vi "DIAdem Parameter CSC.vi"(4 "error in (no error)":errorcluster, 5 "Additional Parameter":string, 6 "Parameter":string, 7 "File Directory":path) -> (0 "error out":errorcluster, 3 "DIAdem Command Parameter":string)   [LabVIEW 2017]
doc: "This VI bundles special additional DIAdem start parameters."
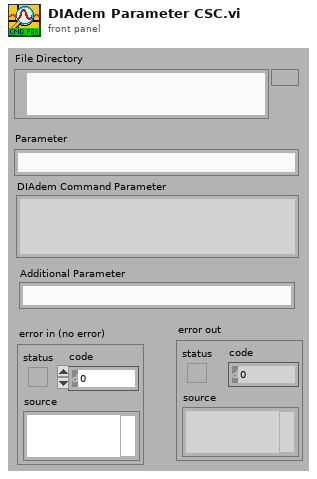
[diagram p1: front panel]
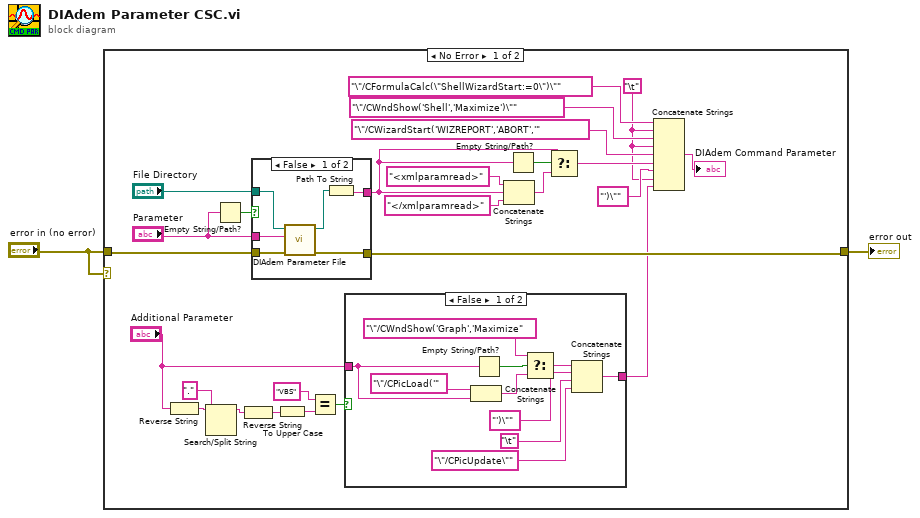
[diagram p0: block diagram]
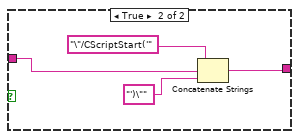
[diagram p2: hidden frame]
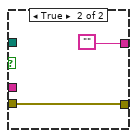
[diagram p3: hidden frame]
diagram:
  n1 = case shown="No Error" "error in (no error)" {
    tunnel: "error in (no error)" -> [w23 w51]
    tunnel: [w22 w51] -> w1
    frame No Error {
      w12 = "\t"
      n2 = Reverse String(1:"Additional Parameter") -> (0:w10:string)
      n3 = Search/Split String(string=w10, search string/char (-)="." ("search char (-)")) -> (substring before match=w9:string)  [unwired: 1 in, 2 out]
      n4 = Empty String/Path?(string/path="Parameter") -> (empty?=w20:bool)
      n5 = Reverse String(1:w9) -> (0:w8:string)
      n6 = case shown="False" w20 {
        tunnel: w23 -> [w48 w50]
        tunnel: [w47 w50] -> w22
        tunnel: "File Directory" -> [w46 _]
        tunnel: "Parameter" -> [w45 _]
        tunnel: [w43 ""] -> w18
        frame False {
          n7 = call <vilib>:"DIAdem Parameter File.vi"("error in (no error)"=w48, "Parameter"=w45, "File Directory"=w46) -> ("error out"=w47:errorcluster, "Parameter File"=w44:path)  [unwired: 3 in]
          n8 = Path To String(path=w44) -> (string=w43:string)
        }
        frame True {
        }
      }
      n9 = To Upper Case(1:w8) -> (0:w7:string)
      n10 = Equal?(x="VBS" ("Substring"), y=w7) -> (x = y?=w4:bool)
      n11 = case shown="False" w4 {
        tunnel: "Additional Parameter" -> [w34 w41]
        tunnel: [w29 w40] -> w3
        frame False {
          n12 = Concatenate Strings("\"/CPicLoad('" ("command"), w34) -> (w36:string)
          n13 = Empty String/Path?(string/path=w34) -> (empty?=w37:bool)
          n14 = Select(t="\"/CWndShow('Graph','Maximize", s=w37, f=w36) -> (s? t:f=w33:string)
          n15 = Concatenate Strings(w33, "')\"" ("Substring"), "\t", "\"/CPicUpdate\"" ("command")) -> (w29:string)
        }
        frame True {
          n16 = Concatenate Strings("\"/CScriptStart('" ("command"), w41, "')\"" ("Substring")) -> (w40:string)
        }
      }
      n17 = Concatenate Strings("<xmlparamread>", w18, "</xmlparamread>") -> (w27:string)
      n18 = Empty String/Path?(string/path=w18) -> (empty?=w26:bool)
      n19 = Select(t=w18, s=w26, f=w27) -> (s? t:f=w17:string)
      n20 = Concatenate Strings("\"/CFormulaCalc(\"ShellWizardStart:=0\")\"" ("DIAdem Command"), w12, "\"/CWndShow('Shell','Maximize')\"", w12, "\"/CWizardStart('WIZREPORT','ABORT','" ("command"), w17, "')\"" ("Substring"), w12, w3) -> (→"DIAdem Command Parameter":string)
    }
    frame Error {
    }
  }
  "error out" <- w1
